vi "fillInGap.vi"(1 "data in":waveform(dbl)[](array[waveform])) -> (0 "data out":waveform(dbl)[](array[waveform]))   [LabVIEW 2017]
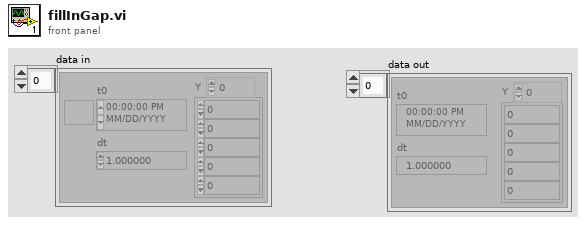
[diagram p1: front panel]
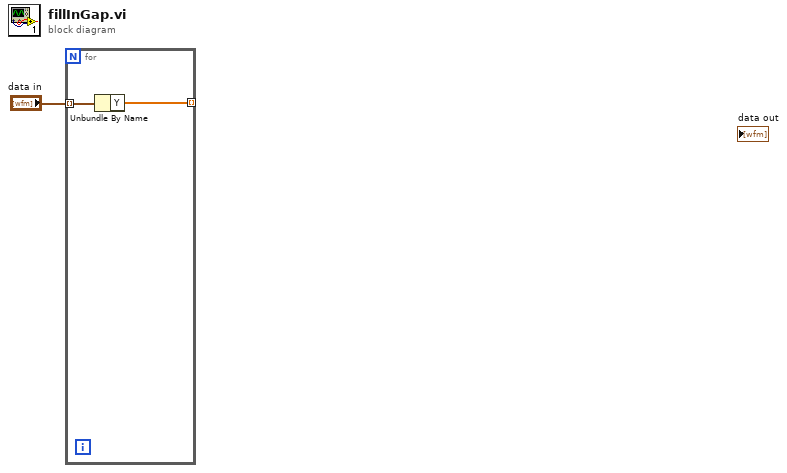
[diagram p0: block diagram]
diagram:
  n1 = for {
    tunnel: "data in" -> [w3] mode=indexing
    tunnel: [w2] -> _ mode=indexing
    n2 = Unbundle By Name(w3) -> ("Y"=w2:dbl[])
  }
